vi "Write Benchmarks.vi"(8 "error in (no error)":errorcluster, 10 "Benchmarks":T1, 11 "CIFCorePlugin in":refnum<class "CIFCorePlugin.lvclass">) -> (0 "error out":errorcluster, 3 "CIFCorePlugin out":refnum<class "CIFCorePlugin.lvclass">)   [LabVIEW 2021, in "CIFCorePlugin.lvclass"]
uses:
  CIFCorePlugin.lvclass
  <vilib>/CIF Foundation/CIF Utilities/Statistics/I64/Stats_I64_CIF_U.lvclass
  Typedef/Benchmarks.ctl
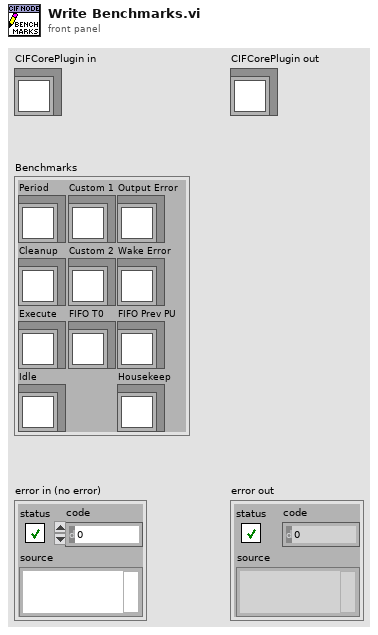
[diagram p1: front panel]
types:
  T1 = typedef "CIFCorePlugin.lvclass/Benchmarks.ctl" = cluster{"Period":refnum<class "Stats_I64_CIF_U.lvclass">, "Wake Error":refnum<class "Stats_I64_CIF_U.lvclass">, "Execute":refnum<class "Stats_I64_CIF_U.lvclass">, "Housekeep":refnum<class "Stats_I64_CIF_U.lvclass">, "Idle":refnum<class "Stats_I64_CIF_U.lvclass">, "Cleanup":refnum<class "Stats_I64_CIF_U.lvclass">, "FIFO T0":refnum<class "Stats_I64_CIF_U.lvclass">, "FIFO Prev PU":refnum<class "Stats_I64_CIF_U.lvclass">, "Output Error":refnum<class "Stats_I64_CIF_U.lvclass">, "Custom 1":refnum<class "Stats_I64_CIF_U.lvclass">, "Custom 2":refnum<class "Stats_I64_CIF_U.lvclass">}
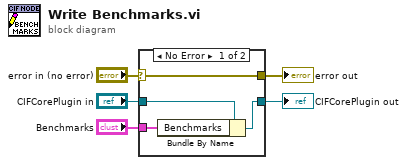
[diagram p0: block diagram]
diagram:
  n1 = case shown="No Error" "error in (no error)" {
    selector: "error in (no error)" -> [w9 w10]
    tunnel: [w9 w10] -> w4
    tunnel: [w7 w11] -> w2
    tunnel: "CIFCorePlugin in" -> [w8 w11]
    tunnel: "Benchmarks" -> [w6 _]
    frame No Error {
      n2 = Bundle By Name(cluster=w8, "Benchmarks"=w6) -> (w7:refnum<class "CIFCorePlugin.lvclass">)
    }
    frame Error {
    }
  }
  "error out" <- w4
  "CIFCorePlugin out" <- w2
